vi "XLP80_Action_BuildMessages_FCCU_Errors.vi"(6 "Init":bool, 8 "err in":errorcluster caption="error", 9 "TimeStamp":dbl format="%.2f") -> (0 "err out":errorcluster caption="error", 2 "Messages":string)   [LabVIEW 2021]
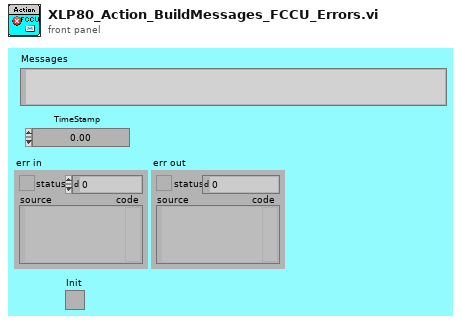
[diagram p1: front panel]
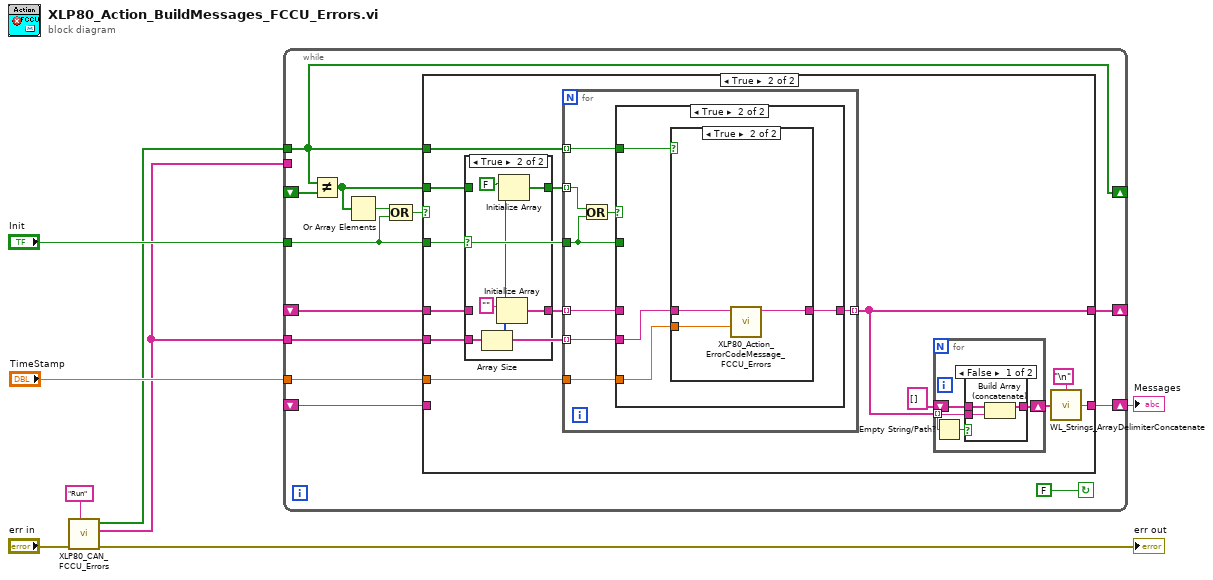
[diagram p0: block diagram]
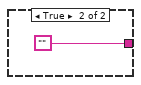
[diagram p4: hidden frame]
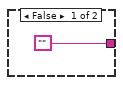
[diagram p5: hidden frame]
diagram:
  n1 = call "XLP80_CAN_FCCU_Errors.vi"("Function"="Run", "err in"="err in") -> ("err out"=→"err out":errorcluster, "FCCU_Names"=w1:string[], "FCCU Errors"=w2:bool[])  [unwired: 7 in]
  n2 = while {
    shift-right: [w12] -> _
    shift-left: _ -> [w14]
    shift-right: [w21] -> _
    shift-left: _ -> [w20]
    shift-right: [w19] -> w8
    shift-left: _ -> [w18]
    tunnel: "Init" -> [w15]
    tunnel: "TimeStamp" -> [w13]
    tunnel: w2 -> [w12]
    tunnel: w1 -> [_]
    tunnel: w1 -> [w9]
    stop <- FALSE continue-if-true
    n3 = Not Equal?(x=w12, y=w14) -> (x != y?=w11:bool[])
    n4 = Or Array Elements(Boolean array=w11) -> (logical OR=w10:bool)
    n5 = Compound Arithmetic op=OR(w10, w15) -> (w16:bool)
    n6 = case shown="True" w16 {
      tunnel: [w22 w26] -> w21
      tunnel: w11 -> [_ w32]
      tunnel: w20 -> [w22 w29]
      tunnel: w12 -> [_ w36]
      tunnel: [w23 w25] -> w19
      tunnel: w15 -> [_ w28]
      tunnel: w18 -> [w23 _]
      tunnel: w13 -> [_ w27]
      tunnel: w9 -> [_ w24]
      frame False {
      }
      frame True {
        n7 = case shown="True" w28 {
          tunnel: w32 -> [w59 _]
          tunnel: [w59 w60] -> w31
          tunnel: [w58 w61] -> w30
          tunnel: w29 -> [w58 _]
          tunnel: w24 -> [_ w62]
          frame False {
          }
          frame True {
            n8 = Array Size(array=w62) -> (size(s)=w65:i32)
            n9 = Initialize Array("", w65) -> (w61:string[])
            n10 = Initialize Array(FALSE, w65) -> (w60:bool[])
          }
        }
        n11 = for {
          tunnel: w36 -> [w44] mode=indexing
          tunnel: w31 -> [w43] mode=indexing
          tunnel: w30 -> [w42] mode=indexing
          tunnel: w28 -> [w41]
          tunnel: [w39] -> w26 mode=indexing
          tunnel: w27 -> [w38]
          tunnel: w24 -> [w37] mode=indexing
          n12 = Or(x=w43, y=w41) -> (x .or. y?=w40:bool)
          n13 = case shown="True" w40 {
            tunnel: [w46 w53] -> w39
            tunnel: w44 -> [_ w52]
            tunnel: w42 -> [w47 _]
            tunnel: w41 -> [w45 _]
            tunnel: w38 -> [_ w51]
            tunnel: w37 -> [_ w50]
            frame False {
              n14 = case shown="False" w45 {
                tunnel: w47 -> [w48 _]
                tunnel: [w48 ""] -> w46
                frame False {
                }
                frame True {
                }
              }
            }
            frame True {
              n15 = case shown="True" w52 {
                tunnel: ["" w57] -> w53
                tunnel: w51 -> [_ w56]
                tunnel: w50 -> [_ w55]
                frame False {
                }
                frame True {
                  n16 = call "XLP80_Action_ErrorCodeMessage_FCCU_Errors.vi"("TimeStamp"=w56, "SYS_Error_Name"=w55) -> ("message string"=w57:string)  [unwired: 9 in]
                }
              }
            }
          }
        }
        n17 = for {
          shift-right: [w67] -> w33
          shift-left: string[] [] -> [w68]
          tunnel: w26 -> [w66] mode=indexing
          n18 = Empty String/Path?(string/path=w66) -> (empty?=w69:bool)
          n19 = case shown="False" w69 {
            tunnel: w68 -> [w72 w73]
            tunnel: [w71 w73] -> w67
            tunnel: w66 -> [w70 _]
            frame False {
              n20 = Build Array (concatenate)(w72, w70) -> (w71:string[])
            }
            frame True {
            }
          }
        }
        n21 = call "WL_Strings_ArrayDelimiterConcatenate.vi"("String Array"=w33, "Delimiter (Tab)"="\n") -> ("String"=w25:string)
      }
    }
  }
  "Messages" <- w8
